vi "nanocal -- nuclear schottky goodness V2.vi"(0 "ζ":dbl(slide)=0.23496699999999998 min=0.0 max=0.3 step=1e-06 scale=0.01..10.0 scale format="%#_3p", 1 "T1":dbl(slide)=0.26762 min=0.0 max=0.3 step=1e-06 scale=0.001..10.0 scale format="%#_3p", 2 "τS":dbl(slide)=0.24445899999999998 min=0.0 max=0.3 step=1e-06 scale=0.001..10.0 scale format="%#_3p", 3 "τN":dbl(slide)=2.349673 min=0.0 max=0.3 step=1e-06 scale=0.001..10.0 scale format="%#_3p", 4 "τC":dbl(slide)=0.0059759999999999995 min=0.0 max=0.3 step=1e-06 scale=0.001..10.0 scale format="%#_3p", 5 "κ0":dbl(slide)=5.58e-10 min=0.0 max=0.3 step=1e-12 scale=1e-10..1e-06 scale format="%#_3p", 7 "ω (rad/sec)":dbl[](array[numeric])=[32012.991918577427, 32390.261658505893, 32466.39798177853, 32499.14340521798, 32517.39286113775, 32529.046092051318, 32537.14525712326, 32543.111142615544, 32547.696343954158, 32551.33675949651, 32554.302325209504, 32556.769142360055, 32558.856995237307, 32560.650202739795, 32562.209843476354, 32563.58125099723, 32564.7987833122, 32565.88895894197, 32566.872575330308, 32567.766175404246, 32568.583086316496, 32569.334166794306, 32570.02835688638, 32570.673085530187, 32571.274580490695, 32571.838104118455, 32572.36813539066, 32572.868514009202, 32573.342552524307, 32573.793126289274, 32574.222746575288, 32574.633618125405, 32575.027687968828, 32575.40668442971, 32575.772149741057, 32576.12546690325, 32576.467883345118, 32576.800529469096, 32577.124435064776, 32577.440543590797, 32577.749724325146, 32578.052781957467, 32578.35046682089, 32578.643482565894, 32578.932492128843, 32579.218126471686, 32579.500987779396, 32579.781656707495, 32580.06069600583, 32580.338656060805, 32580.616078519142, 32580.89350097748, 32581.171461032456, 32581.45050033079, 32581.73116925889, 32582.0140305666, 32582.29966469628, 32582.58867447239, 32582.88169000423, 32583.179375080817, 32583.48243271314, 32583.791613234323, 32584.10772197351, 32584.43162756919, 32584.764273480003, 32585.106690135035, 32585.460007297228, 32585.825472395412, 32586.204468856296, 32586.59853891288, 32587.009410462997, 32587.439030535847, 32587.889604513977, 32588.363642815923, 32588.86402143446, 32589.39405291983, 32589.957576334426, 32590.559071508098, 32591.203800151903, 32591.897990030815, 32592.64907072179, 32593.46598163404, 32594.359581707977, 32595.343197883154, 32596.433373726086, 32597.650906041054, 32599.022313348767, 32600.58195429849, 32602.375161800977, 32604.46301467823, 32606.929831615616, 32609.895397541775, 32613.535812870963, 32618.12101442274, 32624.086899701866, 32632.186064986967, 32643.839295900536, 32662.088751820305, 32694.834175046595, 32770.97049853239], 9 "Voltage out (V)":cdb[](array[numeric])=[1.7183506006211996e-05-0.0001154032788780638i, 1.7124360968751133e-05-0.0001154114779288915i, 1.7049104347380084e-05-0.00011541542942613611i, 1.700437896335042e-05-0.00011541749156201827i, 1.6984579723285106e-05-0.00011542204741013496i, 1.702277369054923e-05-0.00011543195548892015i, 1.713094025845651e-05-0.00011543928112855599i, 1.734249707866828e-05-0.00011543960094139092i, 1.768320429215342e-05-0.0001154245402225022i, 1.8195281152538477e-05-0.00011538335923575508i, 1.8917228661806973e-05-0.00011530288392402138i, 1.9897834564883332e-05-0.00011516640933089982i, 2.154104046962704e-05-0.0001148906117047364i, 2.3247799321765792e-05-0.00011455940834964969i, 2.5364678450551808e-05-0.00011410149936074356i, 2.8645788781885885e-05-0.00011331572480450341i, 3.204749554800641e-05-0.00011242961468546203i, 3.783559691555022e-05-0.00011080033368711338i, 4.245015867332296e-05-0.00010941815048749576i, 4.909131821431355e-05-0.0001073312840925185i, 5.511821898441184e-05-0.00010535829212367013i, 6.178843506022867e-05-0.00010310289174359778i, 7.1079604965352e-05-9.985157907779013e-05i, 7.922304381453334e-05-9.690255343156676e-05i, 8.814778883893872e-05-9.35627973091444e-05i, 9.806709148886077e-05-8.971246458508318e-05i, 0.00011119043245647465-8.437841897470898e-05i, 0.00012253184919712196-7.953180105990741e-05i, 0.00013777724317049346-7.26422052575784e-05i, 0.0001508081004573332-6.638511645494567e-05i, 0.00016547294918783876-5.890291826790314e-05i, 0.00018003847596605868-5.097295421607585e-05i, 0.00019518361086534857-4.2160672625888326e-05i, 0.00021134179818259658-3.207632261667366e-05i, 0.0002372041782935464-1.434566976209705e-05i, 0.00025518143132024254-7.65423157605567e-07i, 0.0002835129702467886+2.297908707067173e-05i, 0.0003060118087631287+4.414715126576145e-05i, 0.00032860772064336976+6.780161699354136e-05i, 0.0003492674091322389+9.188627597766353e-05i, 0.00037498324855458583+0.0001258445655672888i, 0.00040021078021115026+0.00016463936720210011i, 0.00041969942568205823+0.0001996255883353531i, 0.00044367338947118773+0.00025154867300893595i, 0.0004634793607238068+0.0003068834938295352i, 0.00047921028781215815+0.00036805191402776324i, 0.0004880906353641744+0.00042166295770603194i, 0.0004932212623741357+0.0004947057496862386i, 0.000491476456593048+0.0005562791342814882i, 0.000480893803992059+0.0006363872629062725i, 0.0004535995818650303+0.0007373086546111893i, 0.000417087772881063+0.0008226852134031236i, 0.0003564148692854789+0.0009214817173403453i, 0.0003049201646356487+0.0009841224100520793i, 0.00021260191240459413+0.0010684135492785532i, 0.00011714858948470126+0.001130293664798013i, 1.675457544365132e-05+0.0011752384955043165i, -6.8674075405897e-05+0.0012001399159748158i, -0.000156473047607305+0.0012143601357779102i, -0.00026709373934749337+0.0012167952520739987i, -0.0003544271565676041+0.001206585218500233i, -0.00047937600197311275+0.0011721904461218277i, -0.0006086290582260493+0.0011080263068835828i, -0.0007031877411848573+0.0010369948237613604i, -0.0007564526901441745+0.0009845652865779295i, -0.000802489180995596+0.0009292050493656664i, -0.0008414596018105983+0.0008721985101652608i, -0.0008809346482248761+0.0008000538120167723i, -0.0009073902840241921+0.0007382113118499092i, -0.0009264953054508651+0.000680980624166274i, -0.0009405659412141811+0.0006247883223244968i, -0.000951649722530156+0.0005564170049287236i, -0.0009557485581057351+0.0005027508202624884i, -0.0009558464741053665+0.0004515634249715623i, -0.0009509110176922098+0.0003899637122391104i, -0.0009411315169847015+0.00033238768338539245i, -0.0009303400913929496+0.0002890952314710416i, -0.0009171113529290538+0.00024772942260094455i, -0.0009022111527275027+0.00020961974320628598i, -0.0008813746494947608+0.00016554205395646727i, -0.0008581837971946129+0.00012481593212717478i, -0.0008372063466683705+9.328565348151487e-05i, -0.0008165626610594428+6.595676342721183e-05i, -0.0007901155435838691+3.51376371228606e-05i, -0.0007682834352800848+1.2585785624721776e-05i, -0.000746231015527196-7.956667433689733e-06i, -0.0007238798463130141-2.6771164006128246e-05i, -0.0007015567569177018-4.3779400880525094e-05i, -0.000679301954671598-5.9154880569231366e-05i, -0.0006572001413831251-7.301304884663801e-05i, -0.000629855254567978-8.838260380910578e-05i, -0.0006083942229188815-9.917719243438264e-05i, -0.0005768631156754208-0.00011317657292622015i, -0.0005562177438951648-0.00012121832857134644i, -0.0005359092039599222-0.00012831021292074535i, -0.0005145186443378148-0.00013494179211461784i, -0.0004951602053444319-0.00014023403510992087i, -0.00047624970229075174-0.00014478034103386663i, -0.0004577401041527736-0.00014865456703421655i, -0.00043519037796120065-0.00015262867452433312i]) -> (13 "G":dbl=-1.0, 14 "d ln G / d ln ζ":dbl=-1.0, 15 "d ln G / d ln τ1":dbl=-1.0, 16 "d ln G / d ln τS":dbl=-1.0, 17 "d ln G / d ln τN":dbl=-1.0, 18 "d ln G / d ln τC":dbl=-1.0, 19 "d ln G / d ln κ0":dbl=-1.0)   [LabVIEW 2020]
uses:
  3-lorentzian-heat-response action.ctl
panel:
  out "d G / dκ0":dbl=-1.0
  out "d G / dτC":dbl=-1.0
  out "d G / dτN":dbl=-1.0
  out "d G / dτS":dbl=-1.0
  out "d G / dτ1":dbl=-1.0
  out "d G / dζ":dbl=-1.0
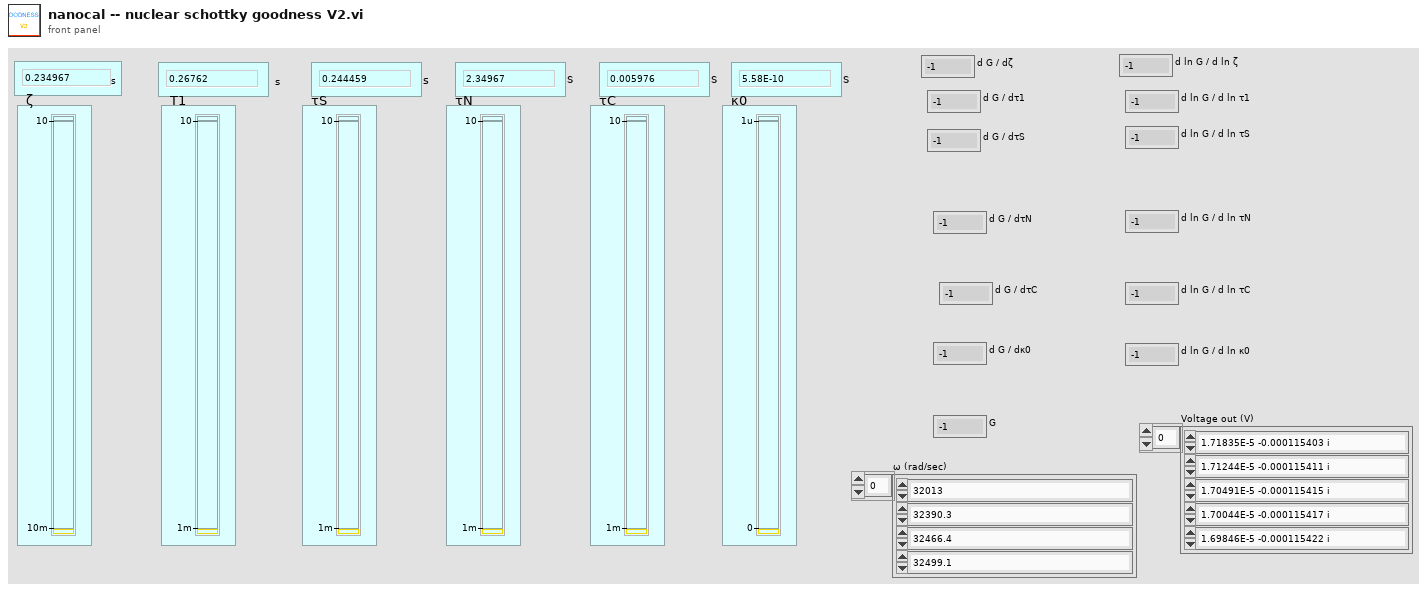
[diagram p1: front panel]
types:
  T1 = typedef "3-lorentzian-heat-response action.ctl" = enum16{"calc R", "create string", "calc m1m2m3", "dζ", "dT1", "dτS", "dτN", "dτC", "d-all", "dκ0"}
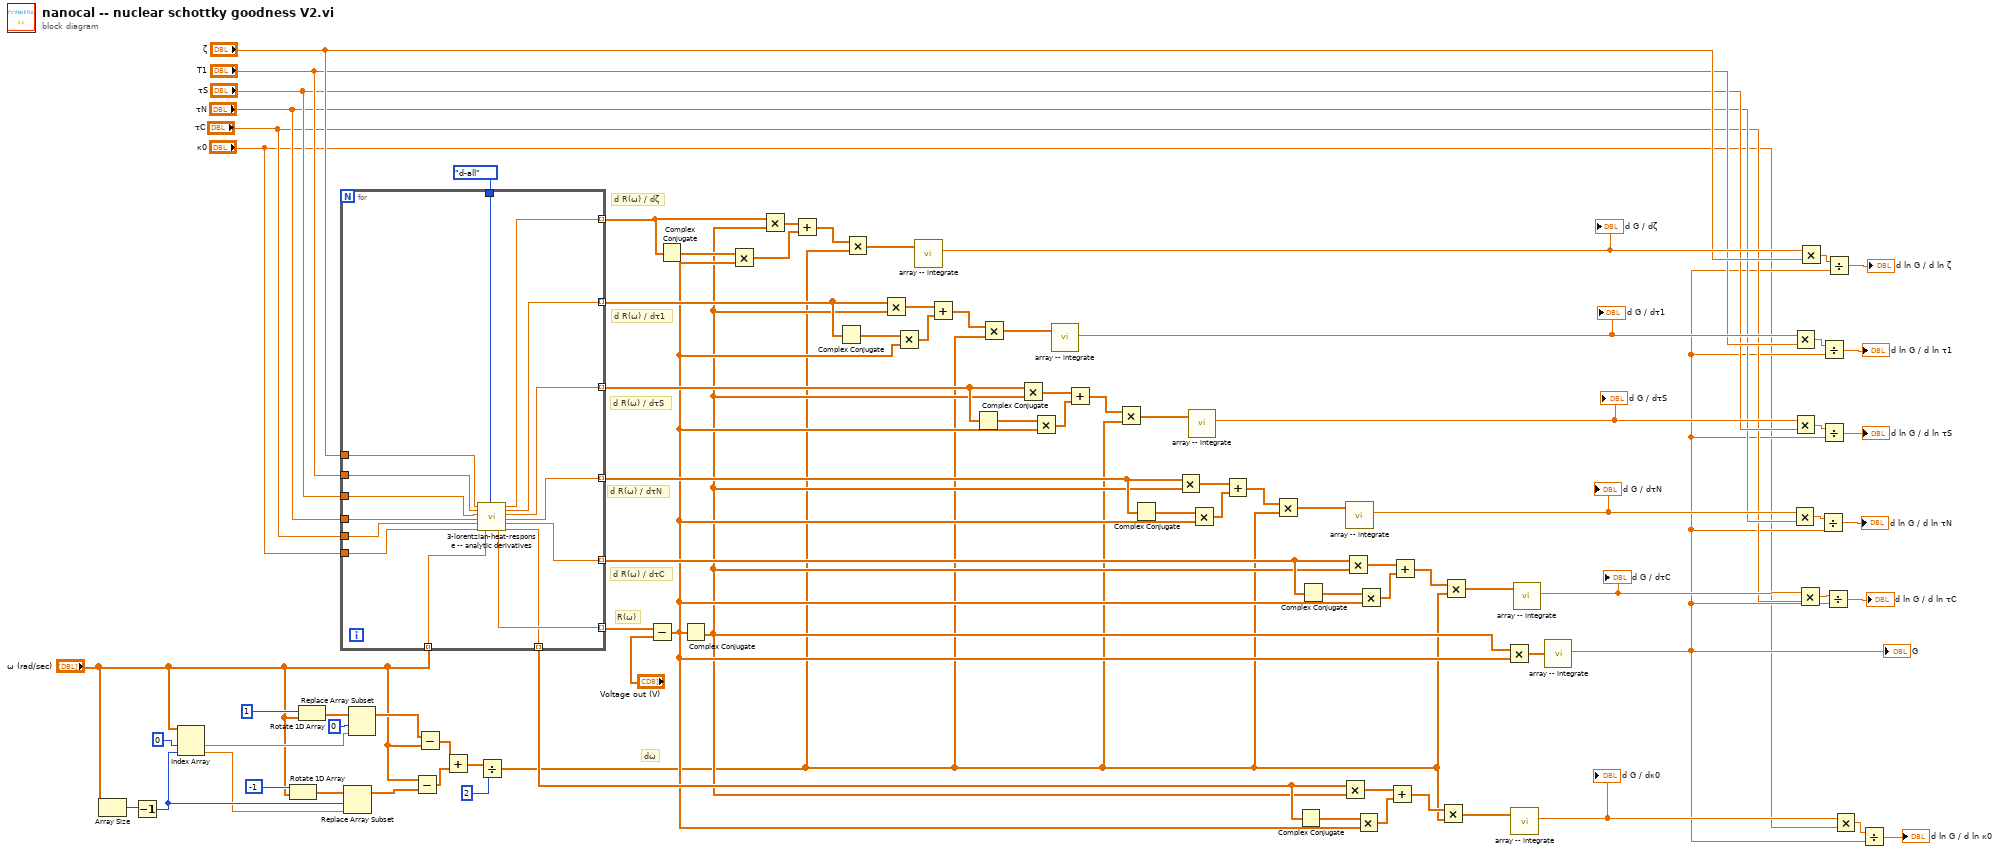
[diagram p0: block diagram]
diagram:
  # "d R(ω) / dτC"
  # "d R(ω) / dτN"
  # "d R(ω) / dτS"
  # "d R(ω) / dτ1"
  # "d R(ω) / dζ"
  # "R(ω)"
  # "dω"
  n1 = Array Size(array="ω (rad/sec)") -> (size(s)=w81:i32)
  n2 = Decrement(x=w81) -> (x-1=w74:i32)
  n3 = Index Array(array="ω (rad/sec)", index #1=0 ("index"), index #2=w74) -> (element #1=w77:dbl, element #2=w73:dbl)
  n4 = Rotate 1D Array(1:"ω (rad/sec)", 2:-1 ("n")) -> (0:w75:dbl[])
  n5 = Rotate 1D Array(1:"ω (rad/sec)", 2:1 ("n")) -> (0:w79:dbl[])
  n6 = for {
    tunnel: "ζ" -> [w100]
    tunnel: "T1" -> [w99]
    tunnel: "τS" -> [w98]
    tunnel: "τN" -> [w97]
    tunnel: "τC" -> [w96]
    tunnel: "κ0" -> [w95]
    tunnel: 3-lorentzian-heat-response_action."d-all" ("action") -> [w91]
    tunnel: "ω (rad/sec)" -> [w94] mode=indexing
    tunnel: [w93] -> w84 mode=indexing
    tunnel: [w92] -> w65 mode=indexing
    tunnel: [w90] -> w53 mode=indexing
    tunnel: [w89] -> w47 mode=indexing
    tunnel: [w88] -> w41 mode=indexing
    tunnel: [w87] -> w35 mode=indexing
    tunnel: [w86] -> w29 mode=indexing
    n7 = call "3-lorentzian-heat-response -- analytic derivatives.vi"("ζ"=w100, "T1"=w99, "τS"=w98, "τN"=w97, "τC"=w96, "κ0"=w95, "ω (rad/sec)"=w94, "action"=w91) -> ("R(ω)"=w93:cdb, "d R(ω) / dζ"=w92:cdb, "d R(ω) /  dT1"=w90:cdb, "d R(ω) /  d τS"=w89:cdb, "d R(ω) /  d τN"=w88:cdb, "d R(ω) /  d τC"=w87:cdb, "d R(ω) /  d κ0"=w86:cdb)  [unwired: 5 in]
  }
  n8 = Replace Array Subset(array=w75, new element=w73, index=w74) -> (w71:dbl[])
  n9 = Replace Array Subset(array=w79, new element=w77, index=0) -> (w72:dbl[])
  n10 = Subtract(x="ω (rad/sec)", y=w71) -> (x-y=w69:dbl[])
  n11 = Subtract(x=w72, y="ω (rad/sec)") -> (x-y=w70:dbl[])
  n12 = Add(x=w70, y=w69) -> (x+y=w68:dbl[])
  n13 = Divide(x=w68, y=2 ("n")) -> (x/y=w26:dbl[])
  n14 = Subtract(x=w84, y="Voltage out (V)") -> (x-y=w28:cdb[])
  n15 = Complex Conjugate(1:w65) -> (0:w64:cdb[])
  n16 = Complex Conjugate(1:w28) -> (0:w27:cdb[])
  n17 = Multiply(x=w64, y=w28) -> (x*y=w62:cdb[])
  n18 = Multiply(x=w65, y=w27) -> (x*y=w63:cdb[])
  n19 = Add(x=w63, y=w62) -> (x+y=w61:cdb[])
  n20 = Complex Conjugate(1:w53) -> (0:w59:cdb[])
  n21 = Multiply(x=w61, y=w26) -> (x*y=w60:cdb[])
  n22 = Multiply(x=w53, y=w27) -> (x*y=w58:cdb[])
  n23 = Multiply(x=w59, y=w28) -> (x*y=w57:cdb[])
  n24 = call "array -- integrate.vi"("Voltage  (V)"=w60) -> ("total"=w25:cdb)  [unwired: 10 in]
  "d G / dζ" <- w25
  n25 = Add(x=w58, y=w57) -> (x+y=w56:cdb[])
  n26 = Complex Conjugate(1:w47) -> (0:w52:cdb[])
  n27 = Multiply(x=w56, y=w26) -> (x*y=w55:cdb[])
  n28 = Multiply(x=w47, y=w27) -> (x*y=w51:cdb[])
  n29 = Multiply(x=w52, y=w28) -> (x*y=w50:cdb[])
  n30 = call "array -- integrate.vi"("Voltage  (V)"=w55) -> ("total"=w19:cdb)  [unwired: 10 in]
  "d G / dτ1" <- w19
  n31 = Add(x=w51, y=w50) -> (x+y=w49:cdb[])
  n32 = Multiply(x=w49, y=w26) -> (x*y=w48:cdb[])
  n33 = Complex Conjugate(1:w41) -> (0:w46:cdb[])
  n34 = Multiply(x=w41, y=w27) -> (x*y=w45:cdb[])
  n35 = call "array -- integrate.vi"("Voltage  (V)"=w48) -> ("total"=w15:cdb)  [unwired: 10 in]
  "d G / dτS" <- w15
  n36 = Multiply(x=w46, y=w28) -> (x*y=w44:cdb[])
  n37 = Add(x=w45, y=w44) -> (x+y=w43:cdb[])
  n38 = Multiply(x=w43, y=w26) -> (x*y=w42:cdb[])
  n39 = Complex Conjugate(1:w29) -> (0:w34:cdb[])
  n40 = Complex Conjugate(1:w35) -> (0:w40:cdb[])
  n41 = Multiply(x=w29, y=w27) -> (x*y=w33:cdb[])
  n42 = Multiply(x=w35, y=w27) -> (x*y=w39:cdb[])
  n43 = call "array -- integrate.vi"("Voltage  (V)"=w42) -> ("total"=w11:cdb)  [unwired: 10 in]
  "d G / dτN" <- w11
  n44 = Multiply(x=w34, y=w28) -> (x*y=w32:cdb[])
  n45 = Multiply(x=w40, y=w28) -> (x*y=w38:cdb[])
  n46 = Add(x=w33, y=w32) -> (x+y=w31:cdb[])
  n47 = Add(x=w39, y=w38) -> (x+y=w37:cdb[])
  n48 = Multiply(x=w31, y=w26) -> (x*y=w30:cdb[])
  n49 = Multiply(x=w37, y=w26) -> (x*y=w36:cdb[])
  n50 = Multiply(x=w27, y=w28) -> (x*y=w54:cdb[])
  n51 = call "array -- integrate.vi"("Voltage  (V)"=w30) -> ("total"=w3:cdb)  [unwired: 10 in]
  "d G / dκ0" <- w3
  n52 = call "array -- integrate.vi"("Voltage  (V)"=w36) -> ("total"=w7:cdb)  [unwired: 10 in]
  "d G / dτC" <- w7
  n53 = call "array -- integrate.vi"("Voltage  (V)"=w54) -> ("total"=w2:cdb)  [unwired: 10 in]
  "G" <- w2
  n54 = Multiply(x=w11, y="τN") -> (x*y=w13:cdb)
  n55 = Multiply(x=w19, y="T1") -> (x*y=w21:cdb)
  n56 = Multiply(x=w15, y="τS") -> (x*y=w17:cdb)
  n57 = Multiply(x=w7, y="τC") -> (x*y=w9:cdb)
  n58 = Multiply(x=w25, y="ζ") -> (x*y=w24:cdb)
  n59 = Divide(x=w13, y=w2) -> (x/y=→"d ln G / d ln τN":cdb)
  n60 = Divide(x=w21, y=w2) -> (x/y=→"d ln G / d ln τ1":cdb)
  n61 = Divide(x=w17, y=w2) -> (x/y=→"d ln G / d ln τS":cdb)
  n62 = Divide(x=w9, y=w2) -> (x/y=→"d ln G / d ln τC":cdb)
  n63 = Divide(x=w24, y=w2) -> (x/y=→"d ln G / d ln ζ":cdb)
  n64 = Multiply(x=w3, y="κ0") -> (x*y=w5:cdb)
  n65 = Divide(x=w5, y=w2) -> (x/y=→"d ln G / d ln κ0":cdb)
